vi "Get Panel Ctl Refnum[].vi"(8 "error in":errorcluster, 11 "Controls[]":refnum<vi>[](array[refnum])) -> (0 "error out":errorcluster, 2 "Controls[] Out":refnum<vi>[](array[refnum]), 3 "Map Out":map{string, refnum<vi>}(c390))   [LabVIEW 2020]
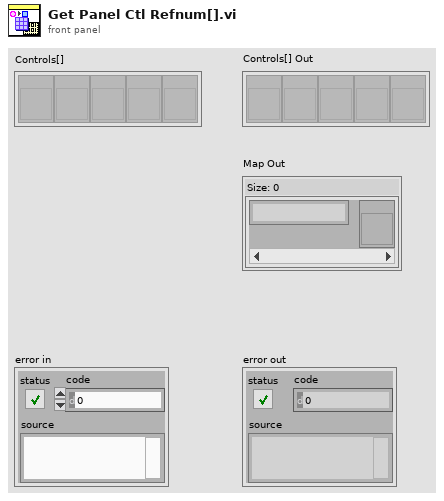
[diagram p1: front panel]
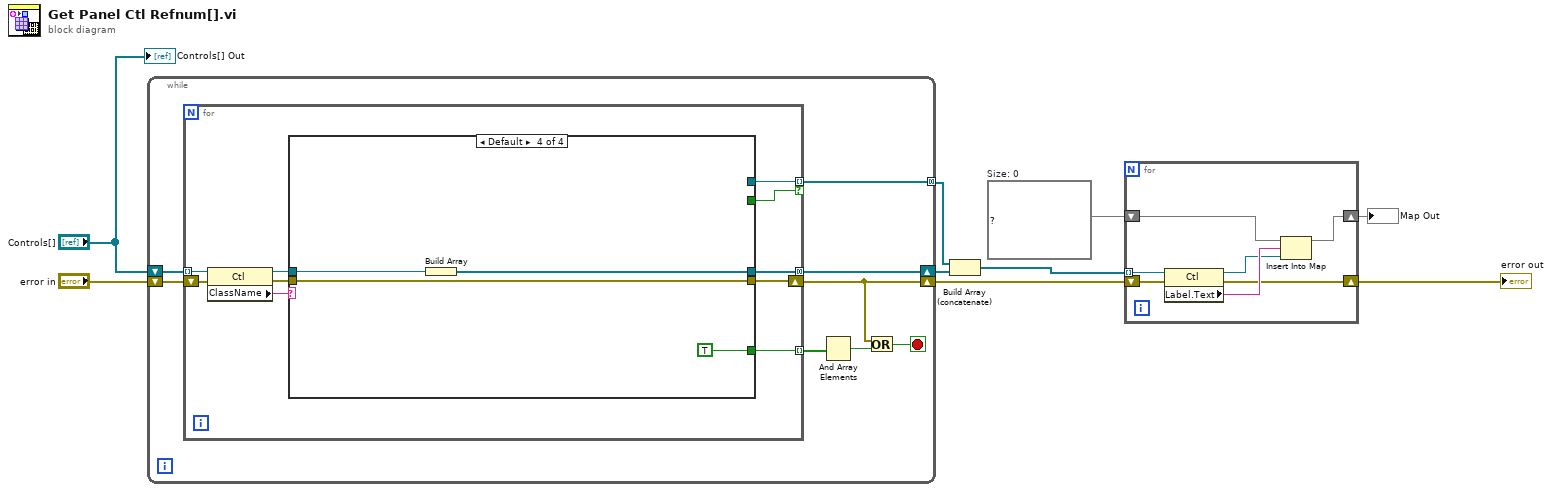
[diagram p0: block diagram]
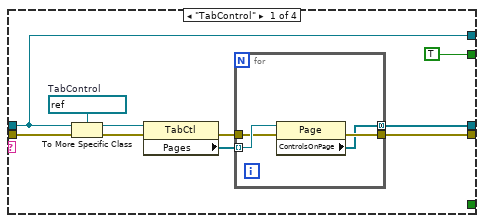
[diagram p2: hidden frame]
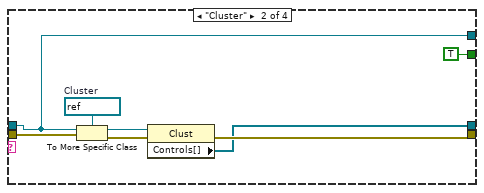
[diagram p3: hidden frame]
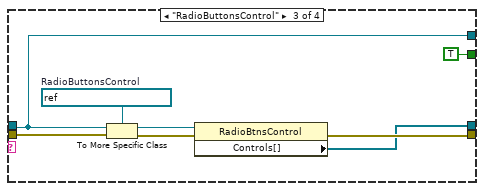
[diagram p4: hidden frame]
diagram:
  w8 = map{string, refnum<vi>} {}  # Size: 0
  n1 = while {
    shift-right: [w12] -> w7
    shift-left: "error in" -> [w16]
    shift-right: [w11] -> w4
    shift-left: "Controls[]" -> [w17]
    tunnel: [w10] -> w5 mode=concatenating
    stop <- w13 stop-if-true
    n2 = for {
      tunnel: w17 -> [w18] mode=indexing
      shift-right: [w23] -> w12
      shift-left: w16 -> [w27]
      tunnel: [w22] -> w11 mode=concatenating
      tunnel: [w21] -> w15 mode=indexing
      tunnel: [w20] -> w10 mode=indexing if=w19
      n3 = property class="Ctl"(reference=w18, error in=w27) -> (reference out=w24:refnum<vi>, error out=w26:errorcluster, "ClassName"=w25:string)
      n4 = case shown="Default" w25 {
        tunnel: w26 -> [w37 w48 w57 w60]
        tunnel: w24 -> [w31 w42 w51 w61]
        tunnel: [w29 w46 w54 w60] -> w23
        tunnel: [w28 w44 w52 w59] -> w22
        tunnel: [_ _ _ TRUE] -> w21
        tunnel: [w31 w42 w51 _] -> w20
        tunnel: [TRUE TRUE TRUE _] -> w19
        frame "TabControl" {
          w36 = refnum<vi> refnum  # TabControl
          n5 = To More Specific Class(target class=w36, reference=w31, error in=w37) -> (specific class reference=w35:refnum<vi>, error out=w34:errorcluster)
          n6 = property class="TabCtl"(reference=w35, error in=w34) -> (error out=w33:errorcluster, "Pages"=w32:refnum<vi>[])  [unwired: 1 out]
          n7 = for {
            tunnel: w33 -> [w40]
            tunnel: w32 -> [w41] mode=indexing
            tunnel: [w39] -> w29
            tunnel: [w38] -> w28 mode=concatenating
            n8 = property class="Page"(reference=w41, error in=w40) -> (error out=w39:errorcluster, "ControlsOnPage"=w38:refnum<vi>[])  [unwired: 1 out]
          }
        }
        frame "Cluster" {
          w49 = refnum<vi> refnum  # Cluster
          n9 = To More Specific Class(target class=w49, reference=w42, error in=w48) -> (specific class reference=w45:refnum<vi>, error out=w47:errorcluster)
          n10 = property class="Clust"(reference=w45, error in=w47) -> (error out=w46:errorcluster, "Controls[]"=w44:refnum<vi>[])  [unwired: 1 out]
        }
        frame "RadioButtonsControl" {
          w55 = refnum<vi> refnum  # RadioButtonsControl
          n11 = To More Specific Class(target class=w55, reference=w51, error in=w57) -> (specific class reference=w53:refnum<vi>, error out=w56:errorcluster)
          n12 = property class="RadioBtnsControl"(reference=w53, error in=w56) -> (error out=w54:errorcluster, "Controls[]"=w52:refnum<vi>[])  [unwired: 1 out]
        }
        frame Default {
          n13 = Build Array(w61) -> (w59:refnum<vi>[])
        }
      }
    }
    n14 = And Array Elements(Boolean array=w15) -> (logical AND=w14:bool)
    n15 = Or(x=w12, y=w14) -> (x .or. y?=w13:bool)
  }
  n16 = Build Array (concatenate)(w5, w4) -> (w6:refnum<vi>[])
  n17 = for {
    tunnel: w6 -> [w68] mode=indexing
    shift-right: [w62] -> w9
    shift-left: w7 -> [w67]
    shift-right: [w63] -> w1
    shift-left: w8 -> [w66]
    n18 = property class="Ctl"(reference=w68, error in=w67) -> (reference out=w64:refnum<vi>, error out=w62:errorcluster, "Label.Text"=w65:string)
    n19 = Insert Into Map(map in=w66, key=w65, value=w64) -> (map out=w63:map{string, refnum<vi>})  [unwired: 2 out]
  }
  "error out" <- w9
  "Map Out" <- w1
  "Controls[] Out" <- "Controls[]"
